vi "ConnectionDataRead.vi"(8 "error in (no error)":errorcluster, 9 "ReadData":refnum<class "ReadData.lvclass">, 10 "Connection":refnum<class "Connection.lvclass">, 11 "CallerMessage in":refnum<class "CallerMessage.lvclass">) -> (0 "error out":errorcluster, 3 "CallerMessage out":refnum<class "CallerMessage.lvclass">)   [LabVIEW 2022 SP3, in "Connection.lvlib" / "CallerMessage.lvclass"]
uses:
  CallerMessage.lvclass
  TcpSocket/Source/TcpSocket/Connection/Connection.lvclass
  ReadData/ReadData.lvclass
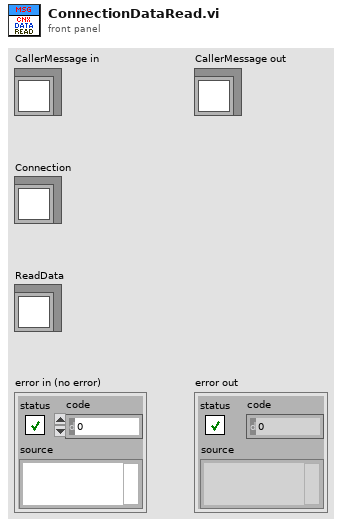
[diagram p1: front panel]
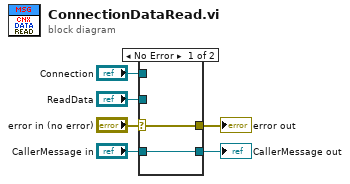
[diagram p0: block diagram]
diagram:
  n1 = case shown="No Error" "error in (no error)" {
    selector: "error in (no error)" -> [w7 w10]
    tunnel: [w7 w10] -> w5
    tunnel: [w8 w9] -> w3
    tunnel: "CallerMessage in" -> [w8 w9]
    tunnel: "Connection" -> [_ _]
    tunnel: "ReadData" -> [_ _]
    frame No Error {
    }
    frame Error {
    }
  }
  "error out" <- w5
  "CallerMessage out" <- w3
